vi "Load Accuracy Test.vi"(8 "error in":errorcluster, 11 "Data In":T1={"Message"="", "Homed?"=FALSE, "NextState"=enum."Timeout", "G.Load"=0.0, "G.Position"=0.0, "Load#"=0, "[G.Loads]"=[], "[TotalLoads]"=[], "[Errors]"=[], "ZeroWait"=0, "Results"=[], "DwellWait"=FALSE, "Test Result"=FALSE, "[CondyleLoads]"=[], "[Max]"=[], "[Min]"=[], "Valid String?"=FALSE, "ScanTime"=timestamp(0 s since 1904-01-01), "ScannedString"="", "LabelDevID"=0, "MfgDate"=timestamp(0 s since 1904-01-01), "[EEPROM Cmds]"=[], "[CalData]"=[], "[A/Ds]"=[], "[A/Dmax]"=[], "[A/Dmin]"=[], "BattMax"=0.0, "BattMin"=0.0, "DwellTime"=2000, "PendingDeviceType"="", "Zero G.load"=0.0, "GAINC Value"="", "Programming Step"=enum."Load EEPROM", "Front Panel Program?"=FALSE, "Final Program?"=FALSE, "PCB Score"=100, "AssyScore"=100, "Pass/Fail #"="", "Result String"="", "Programming Mode"=enum."Initial Program", "Angle Test Step"=enum."Initialize", "Accel Values"=[], "Shutdown Counter"=0, "V1"=0, "V2"=0, "V3"=0, "V4"=0, "EEPROM Data"=[], "Counter"=0, "Page#"=0, "Timer"=timestamp(0 s since 1904-01-01), "Use Mark10?"=FALSE, "Eng-Result#"=0, "DUT Serial #"=0, "Scroll Message?"=FALSE, "Clear Message"=FALSE, "Batt Test Step "=enum."Initialize", "RXTX Window Found?"=FALSE, "Shutdown First Call?"=FALSE, "A2 Delay (msec)"=500, "Support Script"={"Script #"="", "Script Revision"="", "[OEMs]"=[], "[[DeviceTypes]]"=[], "[[DeviceTypesVals]]"=[], "[[List of Errors]]"=[], "Default GAINC"="", "[[ASICtrims]]"=[], "ID For Echo"="", "Condyle A CalFactor"=100, "Condyle B CalFactor"=100, "[OEMs Prefix]"=[], "Packet ID 18"="", "[[Force Table Load Test]]"=[], "[[Force Table AccurTest]]"=[]}, "Serial Table"={"Serial File Path"=path "", "[[Serial Lookup Table]]"=[], "Serial Device Info"=[], "Valid Serial?"=FALSE}, "Target Information"={"Target Brand"="", "Target DeviceType"="", "Target Serial#"=100, "Target Lot#"=0, "Target DevID"=0, "Target Channel"=5}, "Operator"="", "COM Port"="", "Config Path"=path "", "Tx Array"=[], "DUT Parameters"={"Channel"=0, "DeviceID"=0, "Script Rev"=0, "Month"=0, "Day"=0, "Year"=0, "Lot#"=0, "V1"=0, "V2"=0, "V3"=0, "V4"=0, "MFG"=0, "Cal FactorA 10"=0, "Cal FactorB 10  "=0, "Cal FactorA 16"=0, "Cal FactorB 16"=0, "ASICtrim"=[], "TmpChan"=0, "GAINC"="", "Brand"="", "Device"="", "Serial #"=0, "Batt310"=0, "Batt 280"=0}, "FTS Main?"=FALSE, "Loading"={"[Forces]"=[], "[Dwell]"=[], "Loading Step"=enum."Initialize Test"}, "Software Version"="", "Correction Factor"="", "Second Load Test"=FALSE, "Acc Loads"=[], "Mark10 Config"={"H2S%"=[80.0, 85.0, 90.0, 95.0, 100.0], "H2S Speed"=[12.0, 8.0, 6.0, 4.0, 2.0], "H to S"=2.0, "Home Speed"=1.0, "LoadWin"=0.0, "Load Speed"=0.0, "PID"={"Kp"=0.04, "Kd"=0.005001, "Ki"=2.9999999999999923e-05}}, "Channels"={"Transceiver Ch"=5, "Operating Ch"=5, "Start Ch"=0}, "Channel EEPROM"=[], "Load Notes"=[], "Engr Log?"=FALSE, "Time"=[], "Program Retry"=FALSE, "Operator Channel"="", "Target Channel "="", "New Data Program"=FALSE, "NFHU Pass?"=FALSE, "Cycle Number"=0, "Cal Cycle#"=0, "[Avg G.Loads] "=[], "[Avg A/Ds] "=[], "Cal Retry?"=FALSE, "[Total A/Ds]  "=[], "Cycle Num LA"=0, "LA Cycle# "=0, "Shim Num"=0, "Shim#  "=0, "Angle Test?"=FALSE} {"Mark10 Config"."PID"."Ki" min=0.0 max=200.0 format="%.6f"; "Mark10 Config"."PID"."Kd" min=0.0 max=200.0 format="%.6f"; "Mark10 Config"."PID"."Kp" min=0.0 max=200.0 format="%.6f"; "DUT Parameters"."ASICtrim" format="%02x"}) -> (0 "error out":errorcluster, 3 "Data Out":T1={"Message"="", "Homed?"=FALSE, "NextState"=enum."Timeout", "G.Load"=0.0, "G.Position"=0.0, "Load#"=0, "[G.Loads]"=[], "[TotalLoads]"=[], "[Errors]"=[], "ZeroWait"=0, "Results"=[], "DwellWait"=FALSE, "Test Result"=FALSE, "[CondyleLoads]"=[], "[Max]"=[], "[Min]"=[], "Valid String?"=FALSE, "ScanTime"=timestamp(0 s since 1904-01-01), "ScannedString"="", "LabelDevID"=0, "MfgDate"=timestamp(0 s since 1904-01-01), "[EEPROM Cmds]"=[], "[CalData]"=[], "[A/Ds]"=[], "[A/Dmax]"=[], "[A/Dmin]"=[], "BattMax"=0.0, "BattMin"=0.0, "DwellTime"=2000, "PendingDeviceType"="", "Zero G.load"=0.0, "GAINC Value"="", "Programming Step"=enum."Load EEPROM", "Front Panel Program?"=FALSE, "Final Program?"=FALSE, "PCB Score"=100, "AssyScore"=100, "Pass/Fail #"="", "Result String"="", "Programming Mode"=enum."Initial Program", "Angle Test Step"=enum."Initialize", "Accel Values"=[], "Shutdown Counter"=0, "V1"=0, "V2"=0, "V3"=0, "V4"=0, "EEPROM Data"=[], "Counter"=0, "Page#"=0, "Timer"=timestamp(0 s since 1904-01-01), "Use Mark10?"=FALSE, "Eng-Result#"=0, "DUT Serial #"=0, "Scroll Message?"=FALSE, "Clear Message"=FALSE, "Batt Test Step "=enum."Initialize", "RXTX Window Found?"=FALSE, "Shutdown First Call?"=FALSE, "A2 Delay (msec)"=500, "Support Script"={"Script #"="", "Script Revision"="", "[OEMs]"=[], "[[DeviceTypes]]"=[], "[[DeviceTypesVals]]"=[], "[[List of Errors]]"=[], "Default GAINC"="", "[[ASICtrims]]"=[], "ID For Echo"="", "Condyle A CalFactor"=100, "Condyle B CalFactor"=100, "[OEMs Prefix]"=[], "Packet ID 18"="", "[[Force Table Load Test]]"=[], "[[Force Table AccurTest]]"=[]}, "Serial Table"={"Serial File Path"=path "", "[[Serial Lookup Table]]"=[], "Serial Device Info"=[], "Valid Serial?"=FALSE}, "Target Information"={"Target Brand"="", "Target DeviceType"="", "Target Serial#"=100, "Target Lot#"=0, "Target DevID"=0, "Target Channel"=5}, "Operator"="", "COM Port"="", "Config Path"=path "", "Tx Array"=[], "DUT Parameters"={"Channel"=0, "DeviceID"=0, "Script Rev"=0, "Month"=0, "Day"=0, "Year"=0, "Lot#"=0, "V1"=0, "V2"=0, "V3"=0, "V4"=0, "MFG"=0, "Cal FactorA 10"=0, "Cal FactorB 10  "=0, "Cal FactorA 16"=0, "Cal FactorB 16"=0, "ASICtrim"=[], "TmpChan"=0, "GAINC"="", "Brand"="", "Device"="", "Serial #"=0, "Batt310"=0, "Batt 280"=0}, "FTS Main?"=FALSE, "Loading"={"[Forces]"=[], "[Dwell]"=[], "Loading Step"=enum."Initialize Test"}, "Software Version"="", "Correction Factor"="", "Second Load Test"=FALSE, "Acc Loads"=[], "Mark10 Config"={"H2S%"=[80.0, 85.0, 90.0, 95.0, 100.0], "H2S Speed"=[12.0, 8.0, 6.0, 4.0, 2.0], "H to S"=2.0, "Home Speed"=1.0, "LoadWin"=0.0, "Load Speed"=0.0, "PID"={"Kp"=0.04, "Kd"=0.005001, "Ki"=2.9999999999999923e-05}}, "Channels"={"Transceiver Ch"=5, "Operating Ch"=5, "Start Ch"=0}, "Channel EEPROM"=[], "Load Notes"=[], "Engr Log?"=FALSE, "Time"=[], "Program Retry"=FALSE, "Operator Channel"="", "Target Channel "="", "New Data Program"=FALSE, "NFHU Pass?"=FALSE, "Cycle Number"=0, "Cal Cycle#"=0, "[Avg G.Loads] "=[], "[Avg A/Ds] "=[], "Cal Retry?"=FALSE, "[Total A/Ds]  "=[], "Cycle Num LA"=0, "LA Cycle# "=0, "Shim Num"=0, "Shim#  "=0, "Angle Test?"=FALSE} {"Mark10 Config"."PID"."Ki" min=0.0 max=200.0 format="%.6f"; "Mark10 Config"."PID"."Kd" min=0.0 max=200.0 format="%.6f"; "Mark10 Config"."PID"."Kp" min=0.0 max=200.0 format="%.6f"; "DUT Parameters"."ASICtrim" format="%02x"}, 5 "LoadSensors":dbl[](array[numeric]), 7 "Raw Data":u16[](array[numeric]))   [LabVIEW 2015]
uses:
  Controls/LocalVars.ctl
  Controls/Gen2 FT states.ctl
  Controls/Iniial Device Programming.ctl
  ProgramStageControl.ctl
  Controls/Batt Cap Steps.ctl
  Controls/Support Script.ctl
  Controls/Serial Table.ctl
  Controls/Device Information.ctl
  Controls/InfoPacket.ctl
  Controls/Loading.ctl
  Controls/Load Step.ctl
  Controls/Mark10 Config.ctl
  Controls/PID parameters.ctl
  Controls/Channels.ctl
  Controls/Mark10 states.ctl
  Controls/Gen2 FT Globals.vi
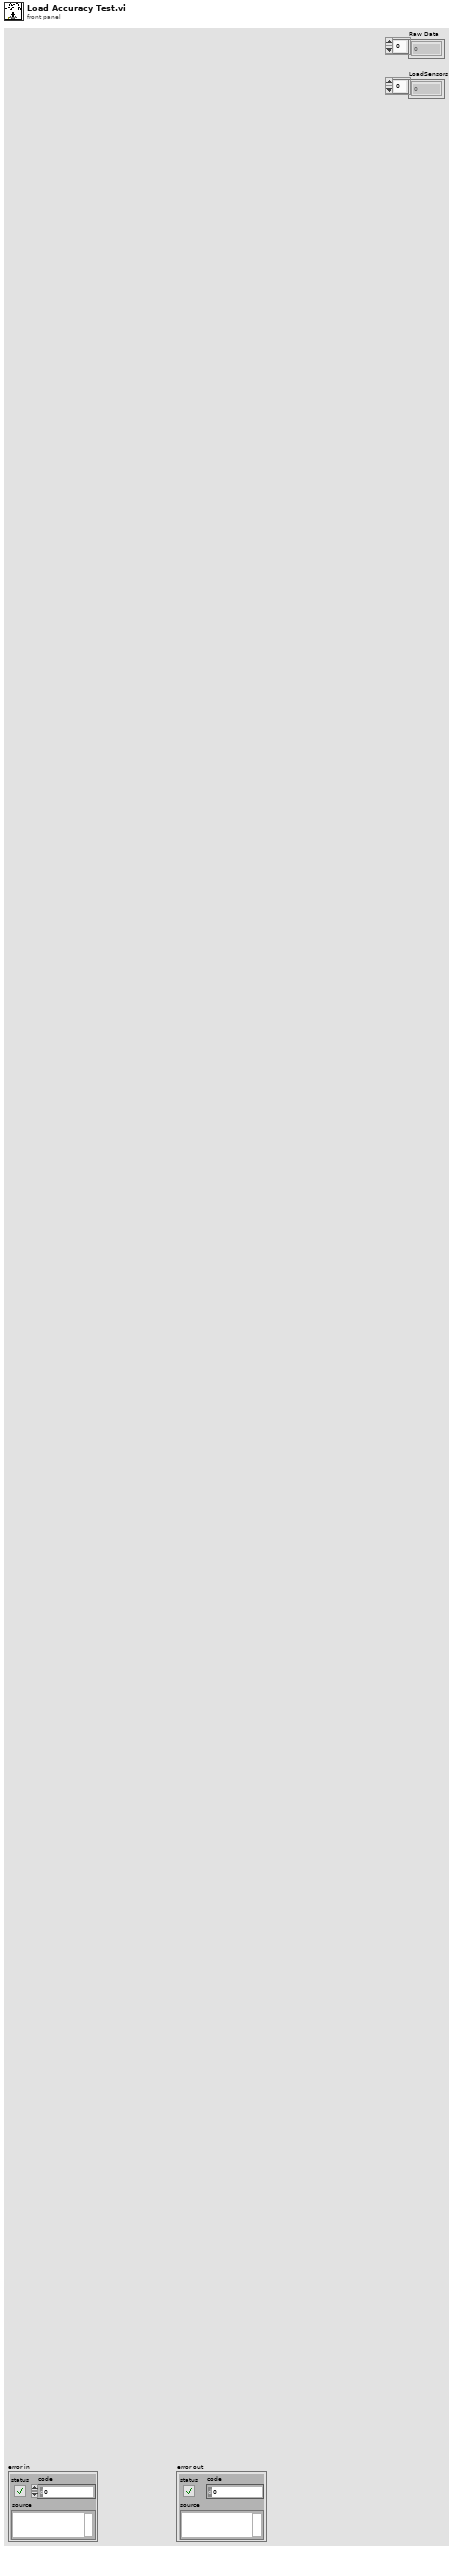
[diagram p1: front panel]
types:
  T1 = typedef "LocalVars.ctl" = cluster{"Message":string, "Homed?":bool, "NextState":T2, "G.Load":dbl, "G.Position":dbl, "Load#":i32, "[G.Loads]":dbl[], "[TotalLoads]":dbl[], "[Errors]":dbl[][], "ZeroWait":u32, "Results":dbl[], "DwellWait":bool, "Test Result":bool, "[CondyleLoads]":dbl[][], "[Max]":dbl[], "[Min]":dbl[], "Valid String?":bool, "ScanTime":timestamp, "ScannedString":string, "LabelDevID":u32, "MfgDate":timestamp, "[EEPROM Cmds]":u8[][], "[CalData]":u8[][], "[A/Ds]":dbl[][], "[A/Dmax]":dbl[], "[A/Dmin]":dbl[], "BattMax":dbl, "BattMin":dbl, "DwellTime":i32, "PendingDeviceType":string, "Zero G.load":dbl, "GAINC Value":string, "Programming Step":T3, "Front Panel Program?":bool, "Final Program?":bool, "PCB Score":i32, "AssyScore":i32, "Pass/Fail #":string, "Result String":string, "Programming Mode":T4, "Angle Test Step":enum16{"Initialize", "Get X", "Get Y", "Get Z", "Next Test"}, "Accel Values":dbl[][], "Shutdown Counter":u32, "V1":i32, "V2":i32, "V3":i32, "V4":i32, "EEPROM Data":i32[][], "Counter":i32, "Page#":i32, "Timer":timestamp, "Use Mark10?":bool, "Eng-Result#":u32, "DUT Serial #":i32, "Scroll Message?":bool, "Clear Message":bool, "Batt Test Step ":T5, "RXTX Window Found?":bool, "Shutdown First Call?":bool, "A2 Delay (msec)":i16, "Support Script":T6, "Serial Table":T7, "Target Information":T8, "Operator":string, "COM Port":string, "Config Path":path, "Tx Array":u8[], "DUT Parameters":T9, "FTS Main?":bool, "Loading":T10, "Software Version":string, "Correction Factor":string, "Second Load Test":bool, "Acc Loads":dbl[][], "Mark10 Config":T12, "Channels":T14, "Channel EEPROM":i32[][], "Load Notes":string[], "Engr Log?":bool, "Time":timestamp[], "Program Retry":bool, "Operator Channel":string, "Target Channel ":string, "New Data Program":bool, "NFHU Pass?":bool, "Cycle Number":i32, "Cal Cycle#":i32, "[Avg G.Loads] ":dbl[], "[Avg A/Ds] ":dbl[][], "Cal Retry?":bool, "[Total A/Ds]  ":dbl[][], "Cycle Num LA":i32, "LA Cycle# ":i32, "Shim Num":i32, "Shim#  ":i32, "Angle Test?":bool}
  T2 = typedef "Gen2 FT states.ctl" = enum16{"---------SETUP-------", "Initialization", "Read Support Data", "Initialize Mark-10", "Initialize Transceiver", "------UTILITIES------", "Change DUT Channel", "Find RxTx Window", "Reset Device", "Scan Channels", "Read Serial Lookup", "Shutdown Device", "ESTOP", "--------USER---------", "Timeout", "-----PROGRAM-----", "Program Device", "------MARK10--------", "Go Home", "MoveUp", "MoveDown", "Goto Load", "Goto Position", "Stop Motor", "---------TESTS--------", "Start Test", "Angle Test", "Load Test", "Load Accuracy Test", "Battery Test", "------RESULTS-------", "End Test", "Display Result", "--------EXIT--------", "Exit"}
  T3 = typedef "Iniial Device Programming.ctl" = enum16{"Load EEPROM", "Send First A1", "Send EEPROM", "Send A1", "Check EEPROM Echo", "Verify transmission", "Programming Successful", "Programming Failed"}
  T4 = typedef "ProgramStageControl.ctl" = enum16{"Initial Program", "GainC", "Scales"}
  T5 = typedef "Batt Cap Steps.ctl" = enum16{"Initialize", "Collect 2.8 Volts", "Collect 3.1 Volts", "Check Results"}
  T6 = typedef "Support Script.ctl" = cluster{"Script #":string, "Script Revision":string, "[OEMs]":string[], "[[DeviceTypes]]":string[][], "[[DeviceTypesVals]]":u16[][], "[[List of Errors]]":string[][], "Default GAINC":string, "[[ASICtrims]]":u8[][], "ID For Echo":string, "Condyle A CalFactor":i32, "Condyle B CalFactor":i32, "[OEMs Prefix]":string[], "Packet ID 18":string, "[[Force Table Load Test]]":dbl[][], "[[Force Table AccurTest]]":dbl[][]}
  T7 = typedef "Serial Table.ctl" = cluster{"Serial File Path":path, "[[Serial Lookup Table]]":string[][], "Serial Device Info":string[], "Valid Serial?":bool}
  T8 = typedef "Device Information.ctl" = cluster{"Target Brand":string, "Target DeviceType":string, "Target Serial#":i32, "Target Lot#":u32, "Target DevID":u32, "Target Channel":u8}
  T9 = typedef "InfoPacket.ctl" = cluster{"Channel":u8, "DeviceID":u32, "Script Rev":u8, "Month":u8, "Day":u8, "Year":u8, "Lot#":u32, "V1":u16, "V2":u16, "V3":u16, "V4":u16, "MFG":u8, "Cal FactorA 10":u8, "Cal FactorB 10  ":u8, "Cal FactorA 16":u8, "Cal FactorB 16":u8, "ASICtrim":u8[], "TmpChan":u8, "GAINC":string, "Brand":string, "Device":string, "Serial #":u64, "Batt310":u16, "Batt 280":u16}
  T10 = typedef "Loading.ctl" = cluster{"[Forces]":dbl[], "[Dwell]":dbl[], "Loading Step":T11}
  T11 = typedef "Load Step.ctl" = enum16{"Initialize Test", "Go Home", "Detect Dev Surface", "Wait to zero Device", "Zero Device", "Do Test", "Test Result"}
  T12 = typedef "Mark10 Config.ctl" = cluster{"H2S%":dbl[], "H2S Speed":dbl[], "H to S":dbl, "Home Speed":dbl, "LoadWin":dbl, "Load Speed":dbl, "PID":T13}
  T13 = typedef "PID parameters.ctl" = cluster{"Kp":dbl, "Kd":dbl, "Ki":dbl}
  T14 = typedef "Channels.ctl" = cluster{"Transceiver Ch":u8, "Operating Ch":u8, "Start Ch":u8}
  T15 = typedef "DeviceInfo.ctl" = cluster{"DevInfo":T9, "Mfg Date":timestamp, "[CalData]":u8[][], "[DevData]":u8[], "GotCal":bool, "CustomCal?":bool, "Packet#":i32}
  T16 = typedef "Mark10 states.ctl" = enum16{"Initialize", "Go Home", "Move Up", "Move Down", "Stop @ Load", "Read Status", "Goto Position", "Goto Device Surface", "Stop Motor", "Shutdown", "Exit"}
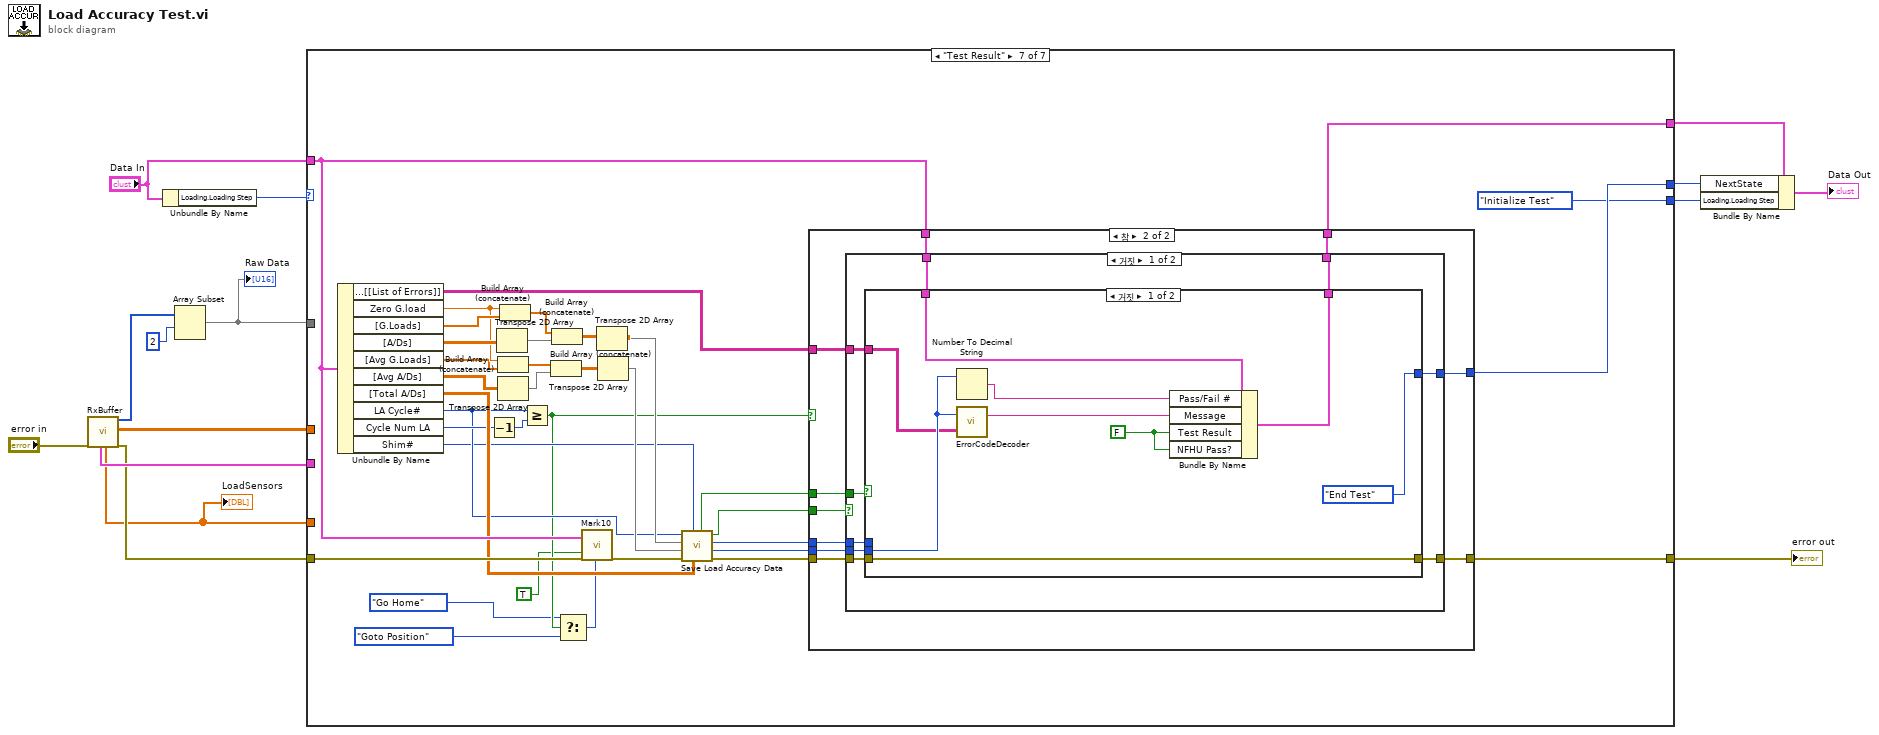
[diagram p0: block diagram]
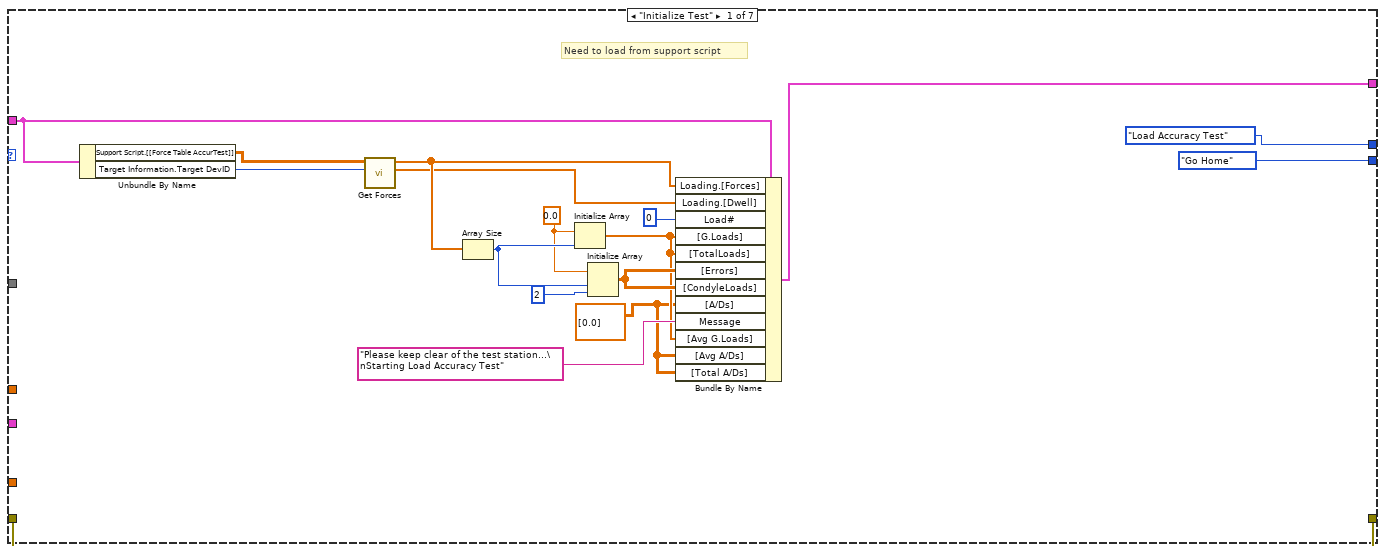
[diagram p2: hidden frame]
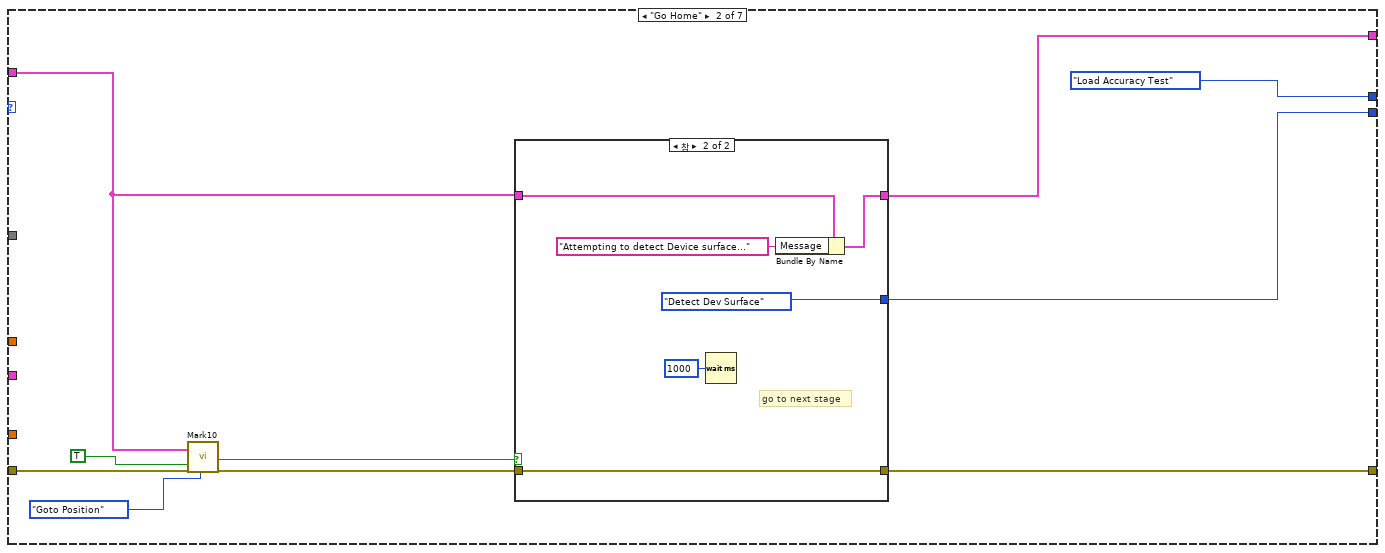
[diagram p3: hidden frame]
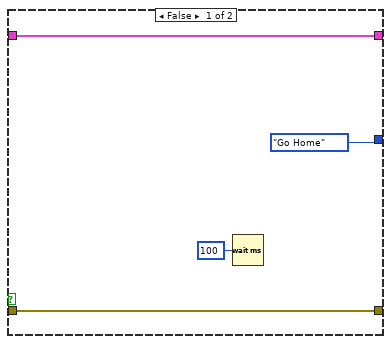
[diagram p4: hidden frame]
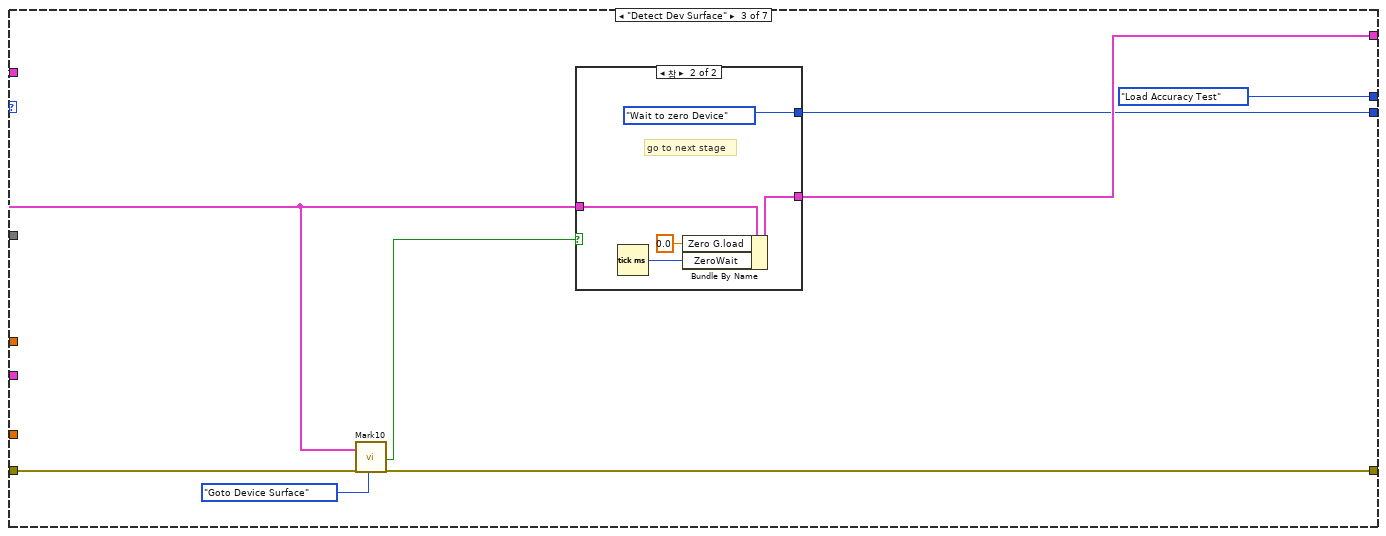
[diagram p5: hidden frame]
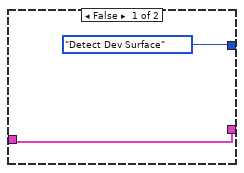
[diagram p6: hidden frame]
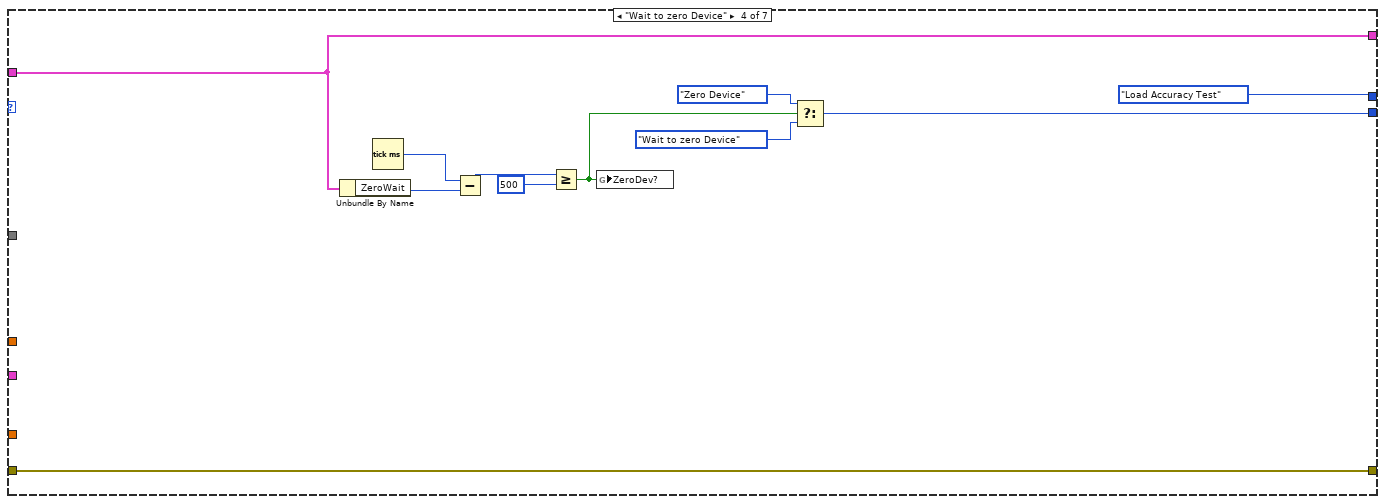
[diagram p7: hidden frame]
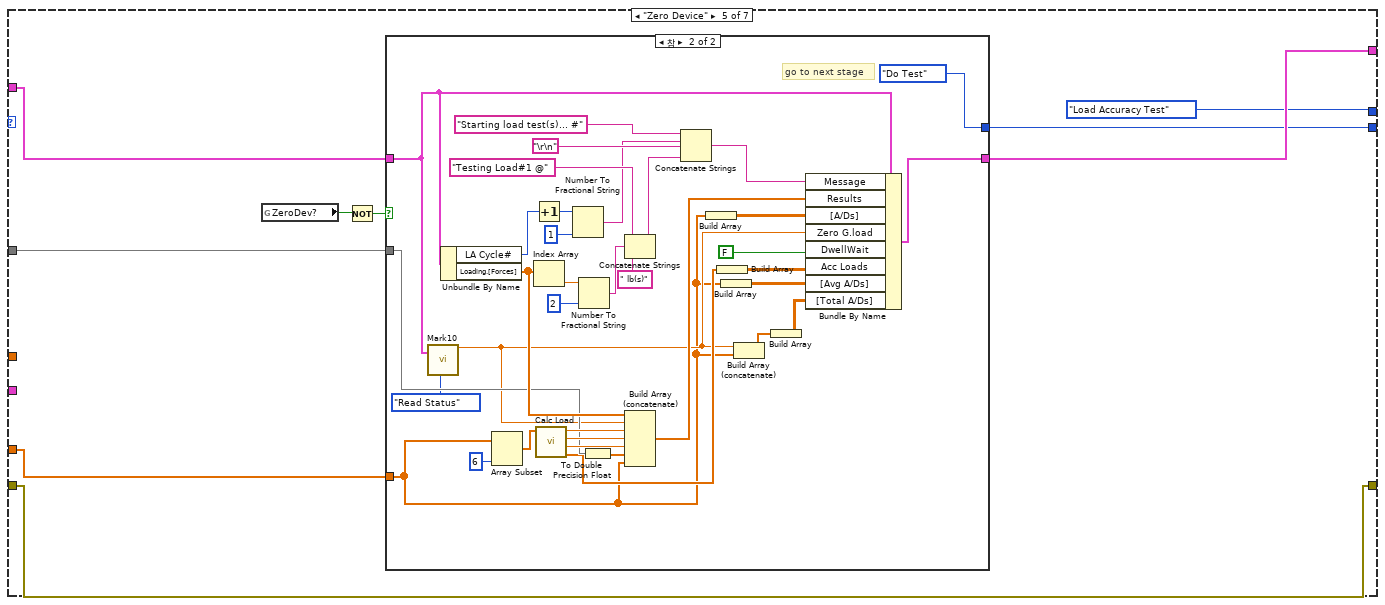
[diagram p8: hidden frame]
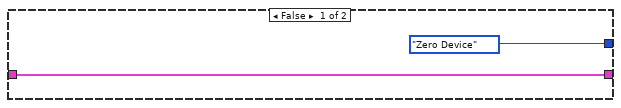
[diagram p9: hidden frame]
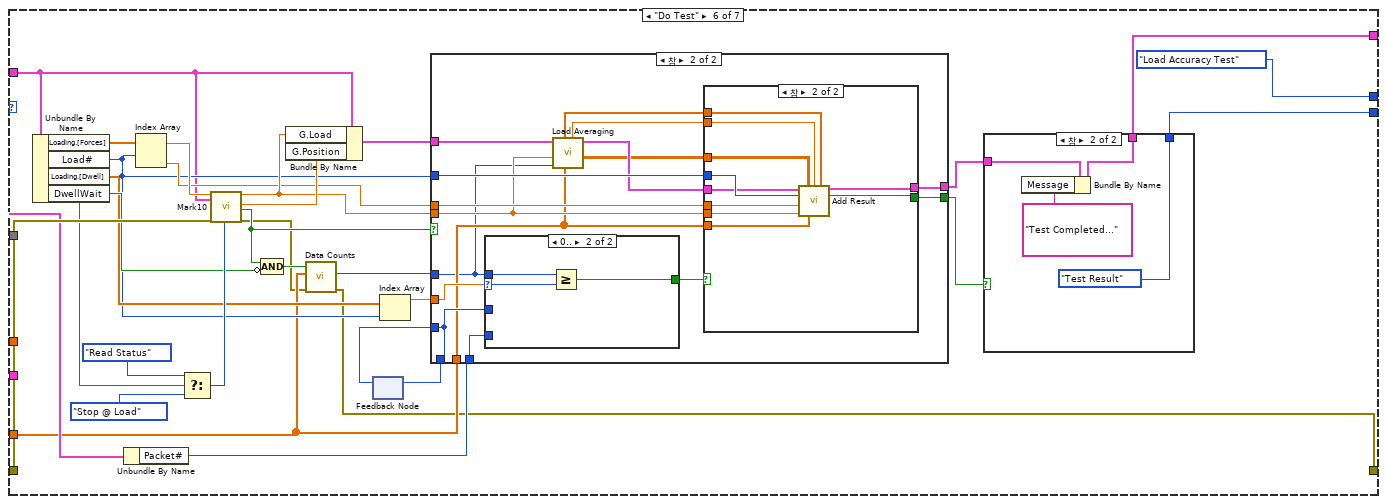
[diagram p10: hidden frame]
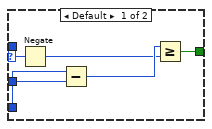
[diagram p12: hidden frame]
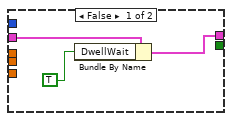
[diagram p13: hidden frame]
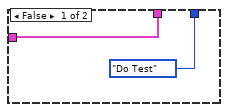
[diagram p14: hidden frame]
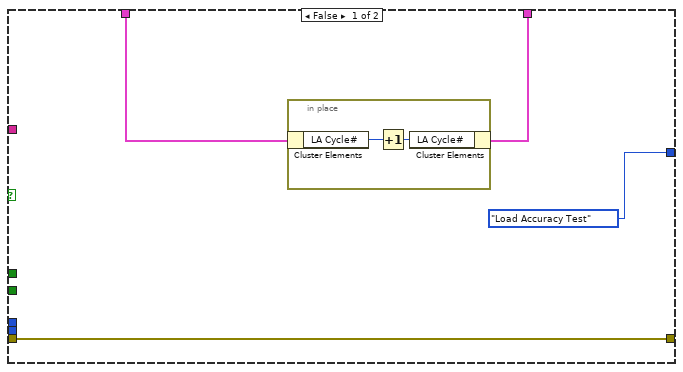
[diagram p15: hidden frame]
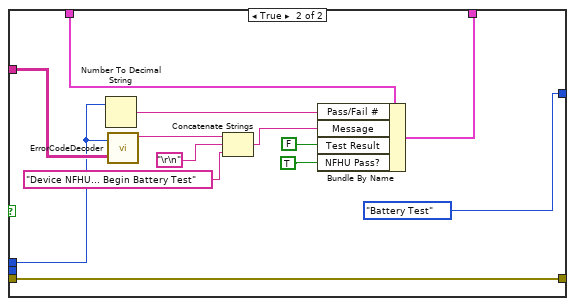
[diagram p16: hidden frame]
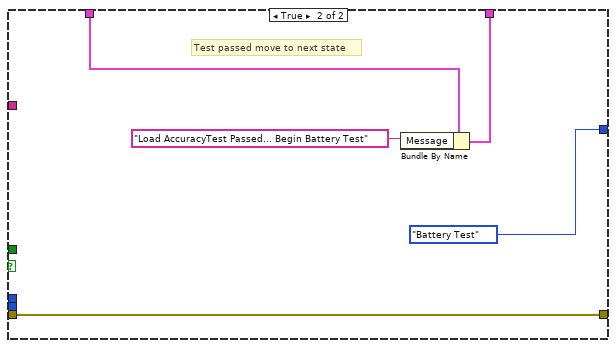
[diagram p17: hidden frame]
diagram:
  n1 = call "RxBuffer.vi"("error in (no error)"="error in") -> ("DeviceParameters"=w12:T15, "LoadSensors"=w1:dbl[], "RxData Out"=w10:u16[], "CalData"=w13:dbl[][], "error out"=w9:errorcluster)  [unwired: 7 in, 7 out]
  "LoadSensors" <- w1
  n2 = Unbundle By Name("Data In") -> ("Loading.Loading Step"=w4:T11)
  n3 = Array Subset(array=w10, index=2) -> (w2:u16[])  [unwired: 1 in]
  "Raw Data" <- w2
  n4 = case shown="\"Test Result\"" w4 {
    tunnel: [Load_Step."Go Home" ("Load Step") w36 w53 w68 w79 w132 Load_Step."Initialize Test" ("Load Step")] -> w3
    tunnel: "Data In" -> [w23 w37 w54 w77 w87 w131 w230]
    tunnel: [w32 w41 w58 w77 w86 w153 w228] -> w6
    tunnel: [w26 w34 w59 w78 w84 w126 w226] -> w7
    tunnel: w9 -> [w26 w42 w60 w78 w84 w154 w236]
    tunnel: w1 -> [_ _ _ _ w82 w128 _]
    tunnel: w2 -> [_ _ _ _ w83 _ _]
    tunnel: w12 -> [_ _ _ _ _ w140 _]
    tunnel: w13 -> [_ _ _ _ _ _ _]
    tunnel: [Gen2_FT_states."Load Accuracy Test" ("NextState") Gen2_FT_states."Load Accuracy Test" ("NextState") Gen2_FT_states."Load Accuracy Test" ("NextState") Gen2_FT_states."Load Accuracy Test" ("NextState") Gen2_FT_states."Load Accuracy Test" ("NextState") Gen2_FT_states."Load Accuracy Test" ("NextState") w229] -> w15
    frame "Initialize Test" {
      w16 = dbl[][] [[0.0]] ("[A/Ds]")
      w29 = 0.0 ("element")
      # "Need to load from support script"
      n5 = Unbundle By Name(w23) -> ("Support Script.[[Force Table AccurTest]]"=w22:dbl[][], "Target Information.Target DevID"=w21:u32)
      n6 = call "Get Forces.vi"("Device ID"=w21, "Force Table"=w22) -> ("Dwell"=w18:dbl[], "Forces"=w19:dbl[])  [unwired: 8 in]
      n7 = Array Size(array=w19) -> (size(s)=w30:i32)
      n8 = Initialize Array(w29, w30) -> (w17:dbl[])
      n9 = Initialize Array(w29, w30, 2 ("dimension size")) -> (w27:dbl[][])
      n10 = Bundle By Name(cluster=w23, "Loading.[Forces]"=w19, "Loading.[Dwell]"=w18, "Load#"=0, "[G.Loads]"=w17, "[TotalLoads]"=w17, "[Errors]"=w27, "[CondyleLoads]"=w27, "[A/Ds]"=w16, "Message"="Please keep clear of the test station...\nStarting Load Accuracy Test", "[Avg G.Loads]"=w17, "[Avg A/Ds]"=w16, "[Total A/Ds]"=w16) -> (w32:T1)
    }
    frame "Go Home" {
      n11 = call "Mark10.vi"("Data In"=w37, "Accuracy \nTest?"=TRUE, "error in (no error)"=w42, "Action"=Mark10_states."Goto Position") -> ("Done?"=w40:bool, "error out"=w35:errorcluster)  [unwired: 11 in, 3 out]
      n12 = case shown="참" w40 {
        tunnel: w37 -> [w46 w51]
        tunnel: [w46 w52] -> w41
        tunnel: [Load_Step."Go Home" ("Load Step") Load_Step."Detect Dev Surface" ("Load Step")] -> w36
        tunnel: w35 -> [w44 w48]
        tunnel: [w44 w48] -> w34
        frame False {
          n13 = Wait (ms)(milliseconds to wait=u32 100) -> ()  [unwired: 1 out]
        }
        frame True {
          # "go to next stage"
          n14 = Wait (ms)(milliseconds to wait=u32 1000) -> ()  [unwired: 1 out]
          n15 = Bundle By Name(cluster=w51, "Message"="Attempting to detect Device surface...") -> (w52:T1)
        }
      }
    }
    frame "Detect Dev Surface" {
      n16 = call "Mark10.vi"("Data In"=w54, "error in (no error)"=w60, "Action"=Mark10_states."Goto Device Surface") -> ("Done?"=w57:bool, "error out"=w59:errorcluster)  [unwired: 12 in, 3 out]
      n17 = case shown="참" w57 {
        tunnel: w54 -> [w62 w66]
        tunnel: [w62 w67] -> w58
        tunnel: [Load_Step."Detect Dev Surface" ("Load Step") Load_Step."Wait to zero Device" ("Load Step")] -> w53
        frame False {
        }
        frame True {
          # "go to next stage"
          n18 = Tick Count (ms)() -> (millisecond timer value=w64:u32)
          n19 = Bundle By Name(cluster=w66, "Zero G.load"=0.0, "ZeroWait"=w64) -> (w67:T1)
        }
      }
    }
    frame "Wait to zero Device" {
      n20 = Unbundle By Name(w77) -> ("ZeroWait"=w75:u32)
      n21 = Tick Count (ms)() -> (millisecond timer value=w76:u32)
      n22 = Subtract(x=w76, y=w75) -> (x-y=w74:u32)
      n23 = Greater Or Equal?(x=w74, y=u32 500) -> (x >= y?=w71:bool)
      n24 = global write "Gen2 FT Globals.vi" "ZeroDev?"(w71) -> ()
      n25 = Select(t=Load_Step."Zero Device" ("Load Step"), s=w71, f=Load_Step."Wait to zero Device" ("Load Step")) -> (s? t:f=w68:T11)
    }
    frame "Zero Device" {
      n26 = global read "Gen2 FT Globals.vi" "ZeroDev?"() -> (w85:bool)
      n27 = Not(x=w85) -> (.not. x?=w81:bool)
      n28 = case shown="참" w81 {
        tunnel: w87 -> [w89 w103]
        tunnel: [w89 w124] -> w86
        tunnel: w82 -> [_ w97]
        tunnel: w83 -> [_ w108]
        tunnel: [Load_Step."Zero Device" ("Load Step") Load_Step."Do Test" ("Load Step")] -> w79
        frame False {
        }
        frame True {
          # "go to next stage"
          n29 = call "Mark10.vi"("Data In"=w103, "Action"=Mark10_states."Read Status") -> ("Live Load"=w98:dbl)  [unwired: 13 in, 4 out]
          n30 = Unbundle By Name(w103) -> ("LA Cycle#"=w94:i32, "Loading.[Forces]"=w115:dbl[])
          n31 = Array Subset(array=w97, length=6) -> (w112:dbl[])  [unwired: 1 in]
          n32 = Increment(x=w94) -> (x+1=w93:i32)
          n33 = Index Array(array=w115) -> (element=w116:dbl)  [unwired: 1 in]
          n34 = call "Calc Load.vi"("[A/D]"=w112) -> ("Loads"=w100:dbl[], "Condyle B Load"=w109:dbl, "Condyle A Load"=w110:dbl, "Total Load"=w111:dbl)  [unwired: 7 in]
          n35 = Number To Fractional String(number=w93, precision (6)=i16 1) -> (F-format string=w91:string)  [unwired: 2 in]
          n36 = Number To Fractional String(number=w116, precision (6)=i16 2) -> (F-format string=w120:string)  [unwired: 2 in]
          n37 = To Double Precision Float(number=w108) -> (double precision float=w107:dbl[])
          n38 = Concatenate Strings("Testing Load#1 @" ("Message"), w120, " lb(s)" ("Message")) -> (w117:string)
          n39 = Build Array (concatenate)(w115, w98, w111, w110, w109, w107, w97) -> (w114:dbl[])
          n40 = Concatenate Strings("Starting load test(s)... #" ("Message"), w91, "\r\n", w117) -> (w118:string)
          n41 = Build Array(w97) -> (w104:dbl[][])
          n42 = Build Array(w100) -> (w101:dbl[][])
          n43 = Build Array(w97) -> (w99:dbl[][])
          n44 = Build Array (concatenate)(w98, w97) -> (w96:dbl[])
          n45 = Build Array(w96) -> (w95:dbl[][])
          n46 = Bundle By Name(cluster=w103, "Message"=w118, "Results"=w114, "[A/Ds]"=w104, "Zero G.load"=w98, "DwellWait"=FALSE, "Acc Loads"=w101, "[Avg A/Ds]"=w99, "[Total A/Ds]"=w95) -> (w124:T1)
        }
      }
    }
    frame "Do Test" {
      n47 = Unbundle By Name(w131) -> ("Loading.[Forces]"=w152:dbl[], "Load#"=w135:i32, "Loading.[Dwell]"=w136:dbl[], "DwellWait"=w141:bool)
      n48 = Unbundle By Name(w140) -> ("Packet#"=w139:i32)
      n49 = Index Array(array=w152, index #1=w135) -> (element #1=w148:dbl, element #2=w147:dbl)  [unwired: 1 in]
      n50 = Select(t=Mark10_states."Read Status" ("Action"), s=w141, f=Mark10_states."Stop @ Load" ("Action")) -> (s? t:f=w142:T16)
      n51 = call "Mark10.vi"("Requested Load"=w148, "Data In"=w131, "error in (no error)"=w154, "Action"=w142) -> ("Live Load"=w149:dbl, "Live Position"=w150:dbl, "Done?"=w146:bool, "error out"=w127:errorcluster)  [unwired: 11 in, 1 out]
      n52 = Compound Arithmetic op=AND(w146, invert w141) -> (w129:bool)
      n53 = Bundle By Name(cluster=w131, "G.Load"=w149, "G.Position"=w150) -> (w151:T1)
      n54 = call "Data Counts.vi"("error in (no error)"=w127, "Data"=w128, "Initialize"=w129) -> ("error out"=w126:errorcluster, "Data Points"=w125:i32)  [unwired: 7 in]
      n55 = feedback #1() -> (w137:i32)  [unwired: 1 in]
      n56 = Index Array(array=w136, index=w135) -> (element=w134:dbl)
      n57 = case shown="참" w146 {
        tunnel: w151 -> [w156 w164]
        tunnel: w135 -> [_ w170]
        tunnel: [_ w172] -> w130
        tunnel: w149 -> [_ w162]
        tunnel: w147 -> [_ w171]
        tunnel: w125 -> [_ w158]
        tunnel: [w156 w169] -> w145
        tunnel: w134 -> [_ w166]
        tunnel: w139 -> [w155 w165]
        tunnel: [w155 w167] -> w138
        tunnel: w137 -> [_ w167]
        tunnel: w128 -> [_ w161]
        frame False {
        }
        frame True {
          n58 = case shown="0.." w166 {
            selector: w166 -> [w174 w179]
            tunnel: w158 -> [_ w181]
            tunnel: [w176 w180] -> w168
            tunnel: w167 -> [w178 _]
            tunnel: w165 -> [w175 _]
            frame Default {
              n59 = Negate(x=w174) -> (-x=w173:i32)
              n60 = Subtract(x=w175, y=w178) -> (x-y=w177:i32)
              n61 = Greater Or Equal?(x=w177, y=w173) -> (x >= y?=w176:bool)
            }
            frame 0.. {
              n62 = Greater Or Equal?(x=w181, y=w179) -> (x >= y?=w180:bool)
            }
          }
          n63 = call "Load Averaging.vi"("Load Sensors"=w161, "Data Points"=w158, "Gauge Load"=w162, "Data In in"=w164) -> ("Total A/D"=w157:dbl[][], "Data In out"=w163:T1, "Average G Load"=w160:dbl, "Average Load Sensors"=w159:dbl[])  [unwired: 4 in]
          n64 = case shown="참" w168 {
            tunnel: w163 -> [w184 w191]
            tunnel: [w183 w194] -> w169
            tunnel: [_ w193] -> w172
            tunnel: w171 -> [_ w189]
            tunnel: w170 -> [_ w192]
            tunnel: w162 -> [_ w190]
            tunnel: w161 -> [_ w188]
            tunnel: w160 -> [_ w187]
            tunnel: w159 -> [_ w186]
            tunnel: w157 -> [_ w185]
            frame False {
              n65 = Bundle By Name(cluster=w184, "DwellWait"=TRUE) -> (w183:T1)
            }
            frame True {
              n66 = call "Add Result.vi"("State-machine Local Variables in"=w191, "Total A/D"=w185, "Avg Live Load"=w187, "[Avg LoadSensors]"=w186, "Load#"=w192, "SetLoad"=w189, "Live Load"=w190, "[LoadSensors]"=w188) -> ("State-machine Local Variables out"=w194:T1, "Done"=w193:bool)  [unwired: 6 in]
            }
          }
        }
      }
      n67 = feedback-in #1(w138) -> ()
      n68 = case shown="참" w130 {
        tunnel: w145 -> [w196 w200]
        tunnel: [w196 w199] -> w153
        tunnel: [Load_Step."Do Test" ("Load Step") Load_Step."Test Result" ("Load Step")] -> w132
        frame False {
        }
        frame True {
          n69 = Bundle By Name(cluster=w200, "Message"="Test Completed...") -> (w199:T1)
        }
      }
    }
    frame "Test Result" {
      n70 = Unbundle By Name(w230) -> ("Support Script.[[List of Errors]]"=w233:string[][], "Zero G.load"=w217:dbl, "[G.Loads]"=w235:dbl[], "[A/Ds]"=w224:dbl[][], "[Avg G.Loads]"=w216:dbl[], "[Avg A/Ds]"=w212:dbl[][], "[Total A/Ds]"=w210:dbl[][], "LA Cycle#"=w207:i32, "Cycle Num LA"=w209:i32, "Shim#"=w206:i32)
      n71 = Decrement(x=w209) -> (x-1=w208:i32)
      n72 = Transpose 2D Array(2D array=w224) -> (transposed array=w222:dbl[][])
      n73 = Build Array (concatenate)(w217, w216) -> (w215:dbl[])
      n74 = Transpose 2D Array(2D array=w212) -> (transposed array=w214:dbl[][])
      n75 = Build Array (concatenate)(w217, w235) -> (w223:dbl[])
      n76 = Greater Or Equal?(x=w207, y=w208) -> (x >= y?=w204:bool)
      n77 = Build Array (concatenate)(w215, w214) -> (w213:dbl[][])
      n78 = Build Array (concatenate)(w223, w222) -> (w221:dbl[][])
      n79 = Select(t=Mark10_states."Go Home" ("Action"), s=w204, f=Mark10_states."Goto Position" ("Action")) -> (s? t:f=w202:T16)
      n80 = call "Mark10.vi"("Data In"=w230, "Accuracy \nTest?"=TRUE, "error in (no error)"=w236, "Action"=w202) -> ("error out"=w234:errorcluster)  [unwired: 11 in, 4 out]
      n81 = Transpose 2D Array(2D array=w221) -> (transposed array=w220:dbl[][])
      n82 = Transpose 2D Array(2D array=w213) -> (transposed array=w211:dbl[][])
      n83 = call "Save Load Accuracy Data.vi"("Total AD Counts"=w210, "Shim #"=w206, "error in (no error)"=w234, "Avg AD Counts"=w211, "AD Counts"=w220, "LA Cycle #"=w207) -> ("error out"=w227:errorcluster, "NFHU Error Code"=w218:i32, "Error Code"=w232:i32, "Pass?"=w231:bool, "NFHU Pass?"=w219:bool)  [unwired: 1 in]
      n84 = case shown="참" w204 {
        tunnel: w233 -> [_ w252]
        tunnel: w232 -> [_ w251]
        tunnel: w231 -> [_ w250]
        tunnel: w230 -> [w239 w249]
        tunnel: [Gen2_FT_states."Load Accuracy Test" ("NextState") w248] -> w229
        tunnel: [w238 w247] -> w228
        tunnel: w227 -> [w240 w246]
        tunnel: [w240 w245] -> w226
        tunnel: w219 -> [_ w244]
        tunnel: w218 -> [_ w243]
        frame False {
          n85 = in-place {
            n86 = in-place-cluster #2(w239) -> ("LA Cycle#"=w242:i32)
            n87 = Increment(x=w242) -> (x+1=w241:i32)
            n88 = in-place-cluster #2("LA Cycle#"=w241) -> (w238:T1)
          }
        }
        frame True {
          n89 = case shown="거짓" w250 {
            tunnel: w252 -> [w261 _]
            tunnel: w251 -> [w260 _]
            tunnel: w249 -> [w259 w287]
            tunnel: [w258 Gen2_FT_states."Battery Test" ("NextState")] -> w248
            tunnel: [w257 w285] -> w247
            tunnel: w246 -> [w256 w288]
            tunnel: [w255 w288] -> w245
            tunnel: w244 -> [w254 _]
            tunnel: w243 -> [w253 _]
            frame False {
              n90 = case shown="거짓" w254 {
                tunnel: w261 -> [w264 w283]
                tunnel: w260 -> [_ w282]
                tunnel: w259 -> [w267 w281]
                tunnel: [Gen2_FT_states."End Test" ("NextState") Gen2_FT_states."Battery Test" ("NextState")] -> w258
                tunnel: [w268 w280] -> w257
                tunnel: w256 -> [w263 w277]
                tunnel: [w263 w277] -> w255
                tunnel: w253 -> [w265 _]
                frame False {
                  w262 = FALSE ("Test Result")
                  n91 = Number To Decimal String(number=w265) -> (decimal integer string=w270:string)  [unwired: 1 in]
                  n92 = call "ErrorCodeDecoder.vi"("array"=w264, "FTS Error Code In"=w265) -> ("Error Message"=w269:string)
                  n93 = Bundle By Name(cluster=w267, "Pass/Fail #"=w270, "Message"=w269, "Test Result"=w262, "NFHU Pass?"=w262) -> (w268:T1)
                }
                frame True {
                  n94 = Number To Decimal String(number=w282) -> (decimal integer string=w279:string)  [unwired: 1 in]
                  n95 = call "ErrorCodeDecoder.vi"("array"=w283, "FTS Error Code In"=w282) -> ("Error Message"=w275:string)
                  n96 = Concatenate Strings(w275, "\r\n", "Device NFHU... Begin Battery Test" ("Message")) -> (w272:string)
                  n97 = Bundle By Name(cluster=w281, "Pass/Fail #"=w279, "Message"=w272, "Test Result"=FALSE, "NFHU Pass?"=TRUE ("Test Result")) -> (w280:T1)
                }
              }
            }
            frame True {
              # "Test passed move to next state"
              n98 = Bundle By Name(cluster=w287, "Message"="Load AccuracyTest Passed... Begin Battery Test") -> (w285:T1)
            }
          }
        }
      }
    }
  }
  "error out" <- w7
  n99 = Bundle By Name(cluster=w6, "NextState"=w15, "Loading.Loading Step"=w3) -> (→"Data Out":T1)
